vi "ykgw.vi"(8 "error in (no error)":errorcluster, 11 "modbusData":refnum<notifier>) -> (0 "error out":errorcluster, 3 "Cluster":T1)   [LabVIEW 2019]
uses:
  instr_dataCluster.ctl
  core/core_autoMonitorDataCluster.ctl
  Instrument.lvclass
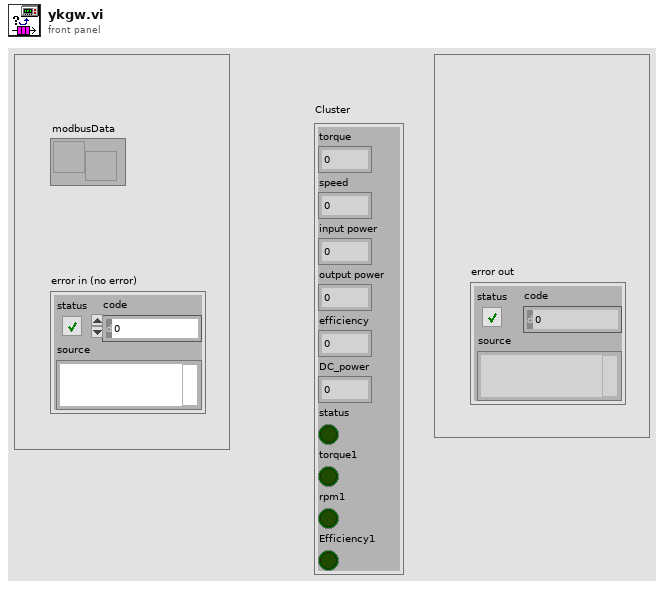
[diagram p1: front panel]
types:
  T1 = typedef "core_autoMonitorDataCluster.ctl" = cluster{"torque":dbl, "speed":dbl, "input power":dbl, "output power":dbl, "efficiency":dbl, "DC_power":dbl, "status":bool, "torque1":bool, "rpm1":bool, "Efficiency1":bool}
  T2 = typedef "Instrument.lvclass/instr_dataCluster.ctl" = cluster{"电源电压 V":dbl, "电源电流A":dbl, "扭矩N/m":dbl, "速度r/M":dbl, "温度℃":dbl[], "流量计L/M":dbl[]}
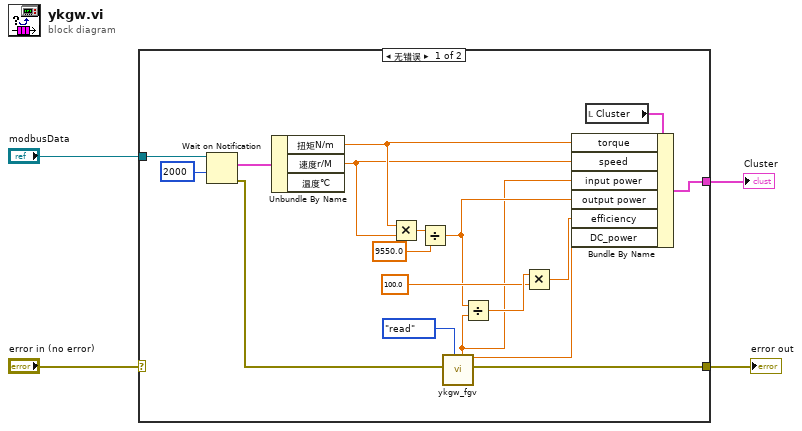
[diagram p0: block diagram]
diagram:
  n1 = case shown="无错误" "error in (no error)" {
    selector: "error in (no error)" -> [_ w23]
    tunnel: [w14 w23] -> w4
    tunnel: "modbusData" -> [w21 _]
    tunnel: [w7 _] -> w1
    frame No Error {
      n2 = Wait on Notification(notifier=w21, timeout in ms (-1)=2000 ("超时毫秒(-1)")) -> (notification=w20:T2, error out=w15:errorcluster)  [unwired: 2 in, 2 out]
      n3 = Unbundle By Name(w20) -> ("扭矩N/m"=w12:dbl, "速度r/M"=w11:dbl)  [unwired: 1 out]
      n4 = Multiply(x=w12, y=w11) -> (x*y=w19:dbl)
      n5 = Divide(x=w19, y=9550.0) -> (x/y=w10:dbl)
      n6 = call "ykgw_fgv.vi"("mode"=enum16{"read", "write"}."read", "error in (no error)"=w15) -> ("error out"=w14:errorcluster, "DC_power"=w5:dbl, "Invertor Output Power"=w9:dbl)  [unwired: 5 in, 2 out]
      n7 = Divide(x=w10, y=w9) -> (x/y=w17:dbl)
      n8 = Multiply(x=w17, y=100.0) -> (x*y=w8:dbl)
      n9 = local read "Cluster"() -> (w13:T1)
      n10 = Bundle By Name(cluster=w13, "torque"=w12, "speed"=w11, "input power"=w9, "output power"=w10, "efficiency"=w8, "DC_power"=w5) -> (w7:T1)
    }
    frame Error {
    }
  }
  "error out" <- w4
  "Cluster" <- w1
